vi "Expand.vi"(8 "error in (no error)":errorcluster, 10 "IB_Tree.lvclass":refnum<class "IB_Tree.lvclass">, 11 "IB_TreeRootItem in":refnum<class "IB_Tree_Item_Proj.lvclass">) -> (0 "error out":errorcluster, 2 "first expansion?":bool, 3 "IB_TreeRootItem out":refnum<class "IB_Tree_Item_Proj.lvclass">)   [LabVIEW 2020, in "IB_Tree_Item_Proj.lvclass"]
uses:
  <vilib>/AppBuilder/IB_Classes/Tree_Item_Proj/IB_Tree_Item_Proj.lvclass
  <vilib>/AppBuilder/IB_Classes/Tree_Item_Proj/IB_Tree_Item_Proj.lvclass/IB_Tree_Item_Proj.ctl
  <vilib>/AppBuilder/IB_Classes/Tree/IB_Tree.lvclass
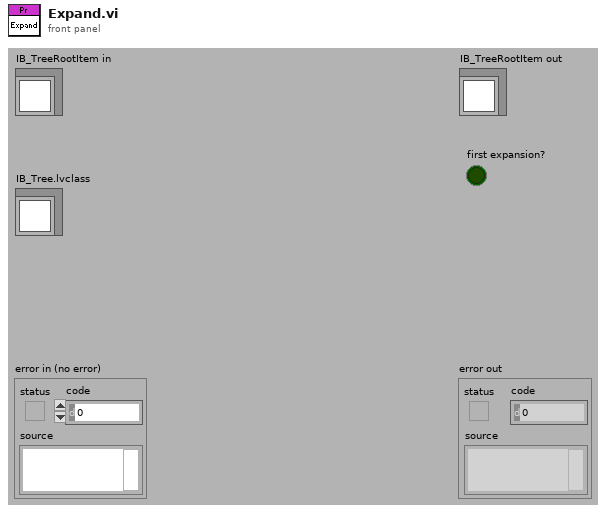
[diagram p1: front panel]
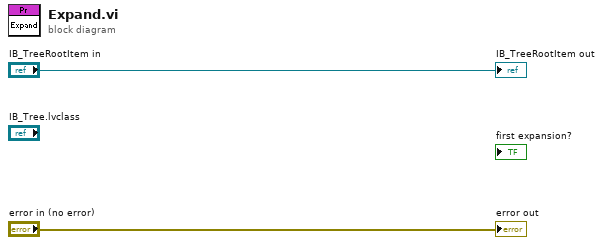
[diagram p0: block diagram]
diagram:
  "error out" <- "error in (no error)"
  "IB_TreeRootItem out" <- "IB_TreeRootItem in"
